vi "Run_ODSS.vi"(7 "Path":path, 8 "error in":errorcluster) -> (0 "error out":errorcluster)   [LabVIEW 2010]
doc: "This Vi implements the routine for executing the simulation in OpenDSS.\n\nCreated by Davis Montenegro\n29-06-2017"
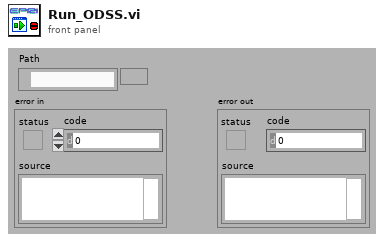
[diagram p1: front panel]
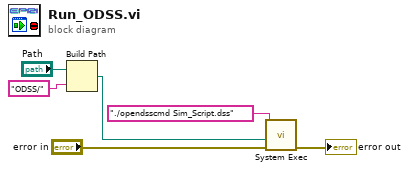
[diagram p0: block diagram]
diagram:
  n1 = Build Path(base path="Path", name or relative path="ODSS/") -> (appended path=w1:path)
  n2 = call <vilib>:"System Exec.vi"("error in (no error)"="error in", "working directory"=w1, "command line"="./opendsscmd Sim_Script.dss") -> ("error out"=→"error out":errorcluster)  [unwired: 5 in, 3 out]
